vi "UDP-test.vi"   [LabVIEW 2019]
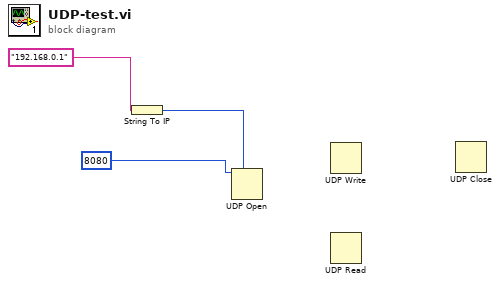
[diagram p0: block diagram]
diagram:
  n1 = String To IP(1:"192.168.0.1") -> (0:w2:u32)
  n2 = UDP Open(7:w2, 11:8080) -> ()  [unwired: 3 in, 3 out]
  n3 = UDP Write() -> ()  [unwired: 6 in, 2 out]
  n4 = UDP Read() -> ()  [unwired: 4 in, 5 out]
  n5 = UDP Close() -> ()  [unwired: 2 in, 2 out]
